vi "Dependency Inspector.vi"() -> (3 "Dependencies Plot":picture)   [LabVIEW 2019, in "DependencyInspector.lvlib"]
uses:
  DependencyInspector.lvlib
  <vilib>/ProgressBar/Progress Bar Dialog.lvclass
panel:
  in  "Open Project":bool
  in  "Include vi.lib":bool
  in  "Projects in Memory":i32(listbox)
  in  "Stop":bool
  in  "Zoom":dbl(slide) scale=0.0..3.0
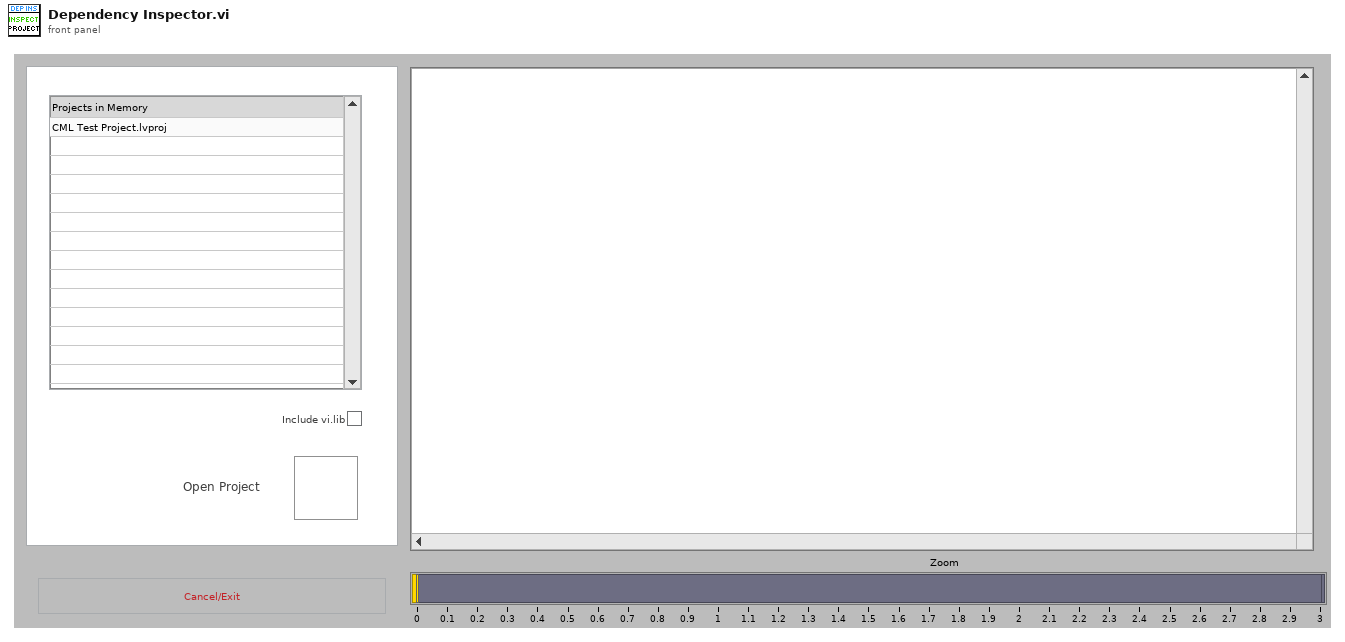
[diagram p1: front panel]
types:
  T1 = typedef "NI_FileType.lvlib/LVFileType.ctl" = enum32{"Invalid file", "Unknown type", "Instrument", "Control", "Polymorphic VI", "Project", "Library", "LVClass", "XControl", "XNode", "Shared library", ".NET assembly", "ActiveX interface", "CIN", "Run-time menu", "Palette menu", "Help file", "LLB", "XNode Edit Dependency", "Class Private Data Control", "Statechart", "MathScript .m file", "Ladder Diagram", "LVLibp", "XNode Build Dependency"}
  T2 = cluster{"path":path, "delimited name":string, "type":T1, "iState":u32, "iStyle":u16, "wStyle":u16, "buttons":u16, "viflags":u32, "viflags2":u32, "links":u32[]}[]
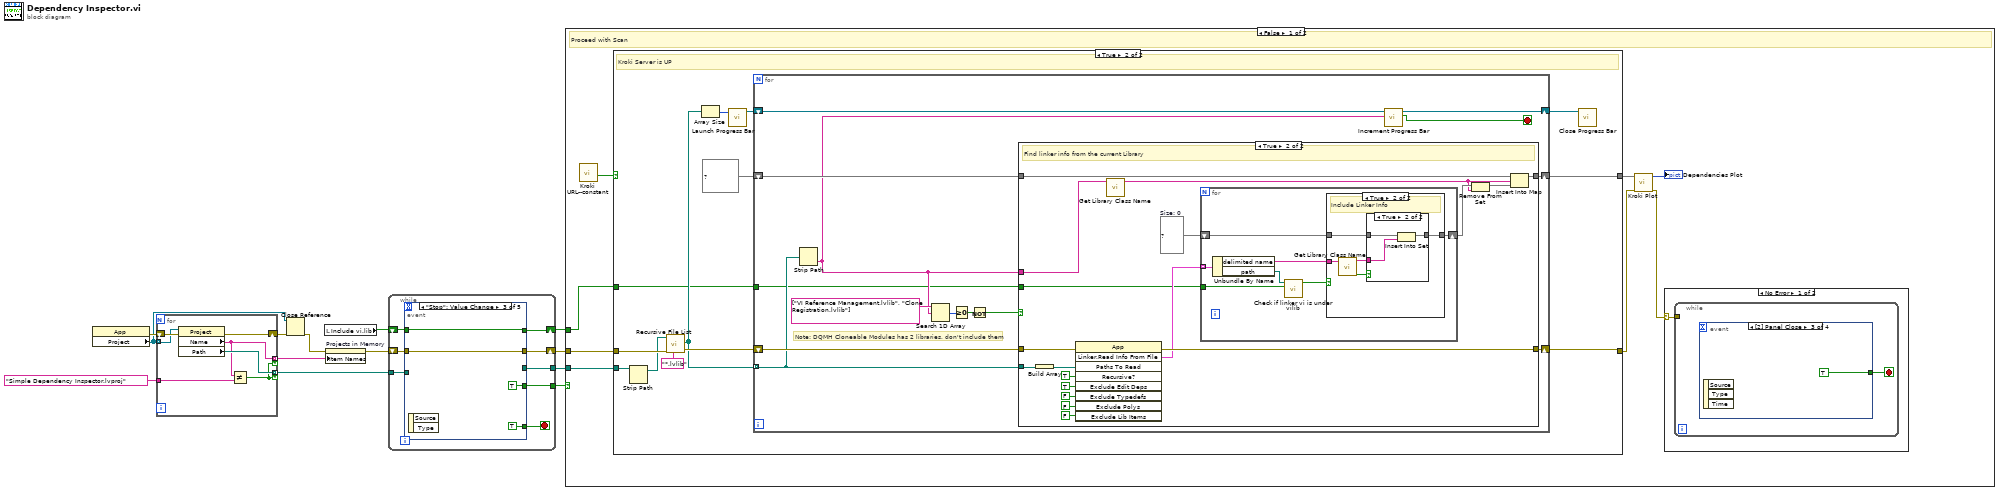
[diagram p0: block diagram]
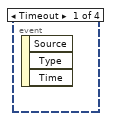
[diagram p6: hidden frame]
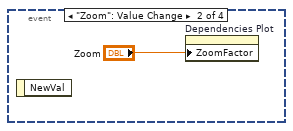
[diagram p7: hidden frame]
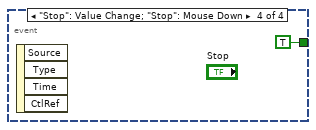
[diagram p8: hidden frame]
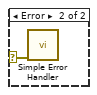
[diagram p9: hidden frame]
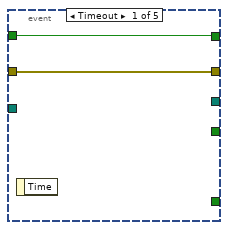
[diagram p11: hidden frame]
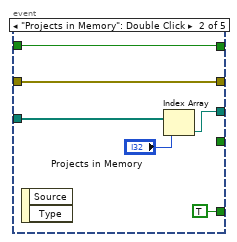
[diagram p12: hidden frame]
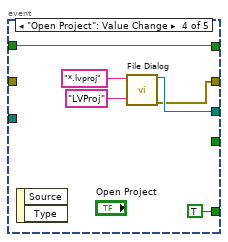
[diagram p13: hidden frame]
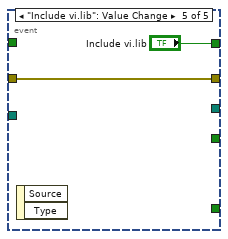
[diagram p14: hidden frame]
diagram:
  n1 = property class="App"() -> (error out=w12:errorcluster, "Project"=w8:refnum<vi>[])  [unwired: 2 in, 1 out]
  n2 = for {
    tunnel: w8 -> [w18] mode=indexing
    tunnel: [w16] -> w7 mode=indexing if=w15
    shift-right: [w20] -> w13
    shift-left: w12 -> [w19]
    tunnel: [w17] -> w6 mode=indexing if=w15
    tunnel: "Simple Dependency Inspector.lvproj" -> [w14]
    n3 = property class="Project"(reference=w18, error in=w19) -> (error out=w20:errorcluster, "Name"=w16:string, "Path"=w17:path)  [unwired: 1 out]
    n4 = Not Equal?(x=w16, y=w14) -> (x != y?=w15:bool)
  }
  n5 = Close Reference(reference=w8, error in (no error)=w13) -> (error out=w11:errorcluster)
  n6 = local read "Include vi.lib"() -> (w1:bool)
  n7 = property on="Projects in Memory" class="LstBox (strict)"(error in=w11, "Item Names"=w7) -> (error out=w10:errorcluster)  [unwired: 1 in, 1 out]
  n8 = while {
    tunnel: w6 -> [w26]
    tunnel: [w25] -> w5
    shift-right: [w27] -> w9
    shift-left: w10 -> [w28]
    shift-right: [w23] -> w4
    shift-left: w1 -> [w22]
    tunnel: [w21] -> w3
    stop <- w24 stop-if-true
    n9 = event shown="[2] \"Stop\": Value Change" {
      selector: _ -> [_ _ _ _ _]
      dyn-events: _ -> [_ _ _ _ _]
      timeout: _ -> [_ _ _ _ _]
      tunnel: w28 -> [w30 w36 w38 _ w48]
      tunnel: [w30 w36 w38 w41 w48] -> w27
      tunnel: w26 -> [_ w35 _ _ _]
      tunnel: [_ w33 _ w43 _] -> w25
      tunnel: [_ TRUE TRUE ("Discard?") TRUE ("Discard?") _] -> w24
      tunnel: [w29 w31 w40 w46 "Include vi.lib"] -> w23
      tunnel: w22 -> [w29 w31 w40 w46 _]
      tunnel: [_ _ TRUE ("Discard?") _ _] -> w21
      event Timeout {
        n10 = event-data() -> ()  [unwired: 1 in, 1 out]
      }
      event "Projects in Memory": Double Click {
        n11 = event-data() -> ()  [unwired: 1 in, 2 out]
        n12 = Index Array(array=w35, index="Projects in Memory") -> (element=w33:path)
      }
      event "Stop": Value Change {
        n13 = event-data() -> ()  [unwired: 1 in, 2 out]
      }
      event "Open Project": Value Change {
        n14 = event-data() -> ()  [unwired: 1 in, 2 out]
        n15 = call "File Dialog"("pattern (all files)"="*.lvproj", "pattern label"="LVProj") -> ("selected path"=w43:path, "error out"=w41:errorcluster)  [unwired: 10 in, 2 out]
      }
      event "Include vi.lib": Value Change {
        n16 = event-data() -> ()  [unwired: 1 in, 2 out]
      }
    }
  }
  n17 = case shown="False" w3 {
    tunnel: w9 -> [w54 _]
    tunnel: w5 -> [w50 _]
    tunnel: w4 -> [w49 _]
    frame False {
      # "Proceed with Scan"
      n18 = call "Kroki URL--constant.vi"() -> ("Server is UP"=w53:bool)  [unwired: 9 in, 2 out]
      n19 = case shown="True" w53 {
        tunnel: w54 -> [w57 w70]
        tunnel: w50 -> [_ w61]
        tunnel: [w57 w68] -> w56
        tunnel: [_ w66] -> w52
        tunnel: w49 -> [_ w58]
        frame False {
        }
        frame True {
          # "Kroki Server is UP"
          n20 = Strip Path(path=w61) -> (stripped path=w62:path)  [unwired: 1 out]
          n21 = call <vilib>:"Recursive File List.vi"("pattern"="*.lvlib", "error in (no error)"=w70, "Folder Path"=w62) -> ("error out"=w69:errorcluster, "All Files in Dir"=w59:path[])  [unwired: 4 in, 3 out]
          n22 = Array Size(array=w59) -> (size(s)=w64:i32)
          n23 = call <vilib>:"Launch Progress Bar.vi"("Total Count"=w64) -> ("Progress Bar Dialog"=w65:refnum<class "Progress Bar Dialog.lvclass">)  [unwired: 9 in, 1 out]
          n24 = for {
            shift-right: [w79] -> w66
            shift-left: map{string, set{string}} {} ("Size: 0") -> [w78]
            shift-right: [w83] -> w68
            shift-left: w69 -> [w84]
            shift-right: [w81] -> w63
            shift-left: w65 -> [w82]
            tunnel: w59 -> [w80] mode=indexing
            tunnel: w58 -> [w71]
            stop <- w77 stop-if-true
            # "Note: DQMH Cloneable Modules has 2 libraries, don't include them"
            n25 = Strip Path(path=w80) -> (name=w73:string)  [unwired: 1 out]
            n26 = Search 1D Array(1D array=string[] ["VI Reference Management.lvlib", "Clone Registration.lvlib"], element=w73) -> (index of element=w75:i32)  [unwired: 1 in]
            n27 = Greater Or Equal To 0?(x=w75) -> (x >= 0?=w76:bool)
            n28 = Not(x=w76) -> (.not. x?=w72:bool)
            n29 = case shown="True" w72 {
              tunnel: w84 -> [w86 w104]
              tunnel: [w86 w103] -> w83
              tunnel: w80 -> [_ w100]
              tunnel: [w85 w97] -> w79
              tunnel: w78 -> [w85 w96]
              tunnel: w73 -> [_ w94]
              tunnel: w71 -> [_ w87]
              frame False {
                # "Not including template libraries"
              }
              frame True {
                w98 = set{string} {}  # Size: 0
                # "Find linker info from the current Library"
                n30 = Build Array(w100) -> (w101:path[])
                n31 = invoke class="App" method="Linker.Read Info From File"(error in=w104, "Paths To Read"=w101, "Recursive?"=TRUE, "Exclude Edit Deps"=TRUE ("Exclude Edit Time Dependencies"), "Exclude Typedefs"=FALSE, "Exclude Polys"=FALSE ("Exclude Poly VIs"), "Exclude Lib Items"=FALSE ("Exclude Unused Library Items")) -> (error out=w103:errorcluster, "Linker.Read Info From File"=w99:T2)  [unwired: 2 in, 7 out]
                n32 = call "Get Library Class Name.vi"("VI In"=w94) -> ("Lib_Class name"=w92:string)  [unwired: 9 in, 1 out]
                n33 = for {
                  tunnel: w99 -> [w111] mode=indexing
                  shift-right: [w108] -> w95
                  shift-left: w98 -> [w109]
                  tunnel: w87 -> [w105]
                  n34 = Unbundle By Name(w111) -> ("delimited name"=w110:string, "path"=w107:path)
                  n35 = call "Check if linker vi is under vilib.vi"("Include VI.lib"=w105, "path"=w107) -> ("Include Info"=w106:bool)  [unwired: 9 in]
                  n36 = case shown="True" w106 {
                    tunnel: w110 -> [_ w117]
                    tunnel: w109 -> [w112 w116]
                    tunnel: [w112 w114] -> w108
                    frame False {
                      # "Do not include Liner Info"
                    }
                    frame True {
                      # "Include Linker Info"
                      n37 = call "Get Library Class Name.vi"("VI In"=w117) -> ("Found?"=w113:bool, "Lib_Class name"=w115:string)  [unwired: 9 in]
                      n38 = case shown="True" w113 {
                        tunnel: w116 -> [w118 w121]
                        tunnel: w115 -> [_ w120]
                        tunnel: [w118 w119] -> w114
                        frame False {
                        }
                        frame True {
                          n39 = Insert Into Set(10:w120, 11:w121) -> (3:w119:set{string})  [unwired: 1 out]
                        }
                      }
                    }
                  }
                }
                n40 = Remove From Set(10:w92, 11:w95) -> (3:w93:set{string})  [unwired: 1 out]
                n41 = Insert Into Map(map in=w96, key=w92, value=w93) -> (map out=w97:map{string, set{string}})  [unwired: 2 out]
              }
            }
            n42 = call <vilib>:"Increment Progress Bar.vi"("Step Name (\"\")"=w73, "Progress Bar Dialog in"=w82) -> ("Cancelled?"=w77:bool, "Progress Bar Dialog out"=w81:refnum<class "Progress Bar Dialog.lvclass">)  [unwired: 7 in, 1 out]
          }
          n43 = call <vilib>:"Close Progress Bar.vi"("Progress Bar Dialog"=w63) -> ()  [unwired: 10 in, 1 out]
        }
      }
      n44 = call "Kroki Plot.vi"("error in"=w56, "Map"=w52) -> ("error out"=w55:errorcluster, "Kroki Plot"=→"Dependencies Plot":picture)  [unwired: 8 in]
      n45 = case shown="No Error" w55 {
        selector: w55 -> [w122 w127]
        frame No Error {
          n46 = while {
            tunnel: w122 -> [_]
            stop <- w123 stop-if-true
            n47 = event shown="[2] Panel Close" {
              selector: _ -> [_ _ _ _]
              dyn-events: _ -> [_ _ _ _]
              timeout: _ -> [_ _ _ _]
              tunnel: [_ _ TRUE ("Discard?") TRUE ("Discard?")] -> w123
              event Timeout {
                n48 = event-data() -> ()  [unwired: 1 in, 3 out]
              }
              event "Zoom": Value Change {
                n49 = event-data() -> ()  [unwired: 1 in, 1 out]
                n50 = property on="Dependencies Plot" class="Pict"("ZoomFactor"="Zoom") -> ()  [unwired: 2 in, 2 out]
              }
              event Panel Close {
                n51 = event-data() -> ()  [unwired: 1 in, 3 out]
              }
              event "Stop": Value Change; "Stop": Mouse Down {
                n52 = event-data() -> ()  [unwired: 1 in, 4 out]
              }
            }
          }
        }
        frame Error {
          n53 = call <vilib>:"Simple Error Handler.vi"("error in (no error)"=w127) -> ()  [unwired: 4 in, 5 out]
        }
      }
    }
    frame True {
      # "User Cancel"
    }
  }
